vi "PID2_GLOBAL.vi"() -> ()   [LabVIEW 2018]
panel:
  in  "PID2 GLOBAL":dbl
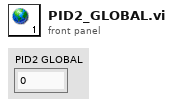
[diagram p1: front panel]
diagram:
